vi "SVPO TDMS Write SGL Array (N Ch 1 Info).vi"(0 "tdms file":refnum<k34>, 1 "write channel properties? (T)":bool=TRUE, 5 "group name in":string="Waveform", 7 "channel names in":string[](array[string]), 9 "scaled signals [EU]":sgl[][](array[numeric]), 11 "sampling rate [Hz]":dbl=1.0, 12 "unit label":string) -> (4 "tdms file out":refnum<k34>, 6 "group name out":string, 8 "channel names out":string[](array[string]))   [LabVIEW 2017]
doc: "Writes single-precision waveform or scaled array data to the specified .tdms file in a format specific to the polymorphic instance. Use this VI on embedded targets that have limited computational resources. Wire data to the <B>scaled signal [EU]</B> input to determine the polymorphic instance to use or manually select the instance."
uses:
  <vilib>/addons/_NISVFA/_Shared subVIs/Controls/svc_X-Axis Units.ctl
  <vilib>/addons/_NISVFA/_Shared subVIs/Controls/NI Channel Properties.ctl
  <vilib>/addons/_NISVFA/_Shared subVIs/Controls/LV Datatypes.ctl
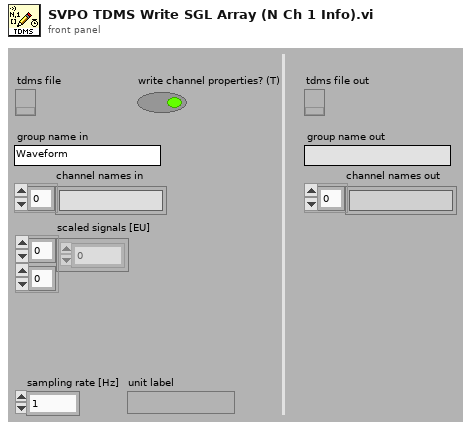
[diagram p1: front panel]
types:
  T1 = typedef "NI Channel Properties.ctl" = u16
  T2 = typedef "LV Datatypes.ctl" = i32
  T3 = typedef "svc_X-Axis Units.ctl" = u16
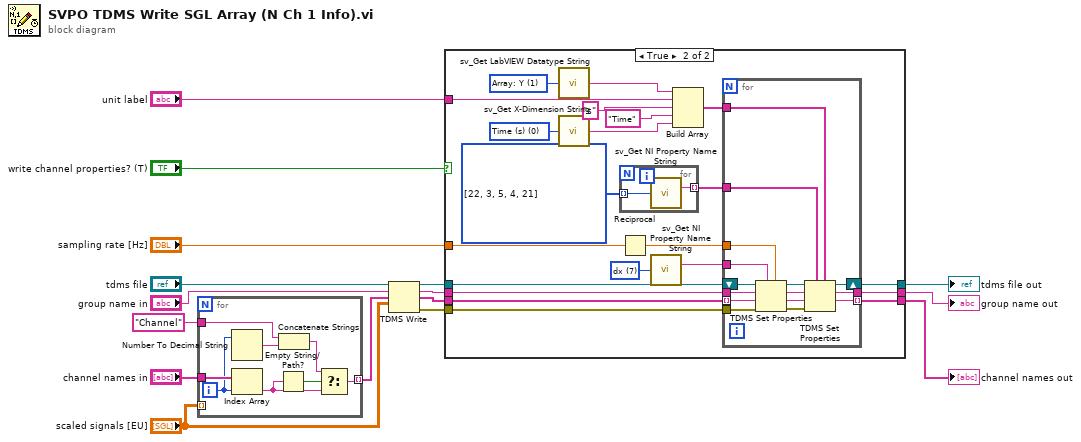
[diagram p0: block diagram]
diagram:
  n1 = for {
    tunnel: "channel names in" -> [w24]
    tunnel: [w23] -> w6 mode=indexing
    tunnel: "Channel" ("string") -> [w17]
    tunnel: "scaled signals [EU]" -> [_] mode=indexing
    i -> [w20]
    n2 = Number To Decimal String(number=w20) -> (decimal integer string=w19:string)  [unwired: 1 in]
    n3 = Index Array(array=w24, index=w20) -> (element=w21:string)
    n4 = Empty String/Path?(string/path=w21) -> (empty?=w22:bool)
    n5 = Concatenate Strings(w17, w19) -> (w18:string)
    n6 = Select(t=w18, s=w22, f=w21) -> (s? t:f=w23:string)
  }
  n7 = TDMS Write(0:"tdms file", 5:"group name in", 7:w6, 9:"scaled signals [EU]") -> (4:w15:refnum<k34>, 6:w13:string, 8:w12:string[], 15:w1:errorcluster)  [unwired: 2 in]
  n8 = case shown="True" "write channel properties? (T)" {
    tunnel: [w27 w41] -> w10
    tunnel: w12 -> [w25 w46]
    tunnel: w13 -> [w26 w45]
    tunnel: w15 -> [w27 w44]
    tunnel: [w26 w48] -> w9
    tunnel: [w25 w42] -> w4
    tunnel: "sampling rate [Hz]" -> [_ w38]
    tunnel: "unit label" -> [_ w34]
    tunnel: w1 -> [_ w36]
    frame False {
    }
    frame True {
      w28 = T1[] [22, 3, 5, 4, 21] items=["Channel name", "Channel description", "Y-axis label", "Y-axis unit string", "X-axis label", "X-axis unit string", "x0", "dx", "Number of samples", "X channel", "Filter settled", "dB reference", "Window", "Window parameter", "Window size", "FFT size", "Peak units", "Spectrum type", "Magnitude scale", "Spectral density", "Sensor sensitivity (mV/EU)", "X-axis domain", "LabVIEW datatype"]
      w47 = T2 1 items=["String"=-2, "Boolean"=-1, "Scalar: y"=0, "Array: Y"=1, "Waveform: t0, dt, Y, variant"=2, "Cluster: x0, dx, Y"=3, "Cluster: X, Y"=4, "Waterfall"=5, "Colormap"=6] ("LabVIEW datatype")
      w39 = T1 7 items=["Channel name", "Channel description", "Y-axis label", "Y-axis unit string", "X-axis label", "X-axis unit string", "x0", "dx", "Number of samples", "X channel", "Filter settled", "dB reference", "Window", "Window parameter", "Window size", "FFT size", "Peak units", "Spectrum type", "Magnitude scale", "Spectral density", "Sensor sensitivity (mV/EU)", "X-axis dimension", "LabVIEW datatype", "Function type", "Function subtype"] ("property")
      w43 = T3 0 items=["Time (s)"=0, "Frequency-CB (Hz)"=1, "Frequency-CPB (Hz)"=1248, "Frequency-Arbitrary (Hz)"=2357, "Quefrency (s)"=2, "Revolutions (rev)"=3, "Order"=4, "Speed (RPM)"=11, "Speed (rad/s)"=21, "Index"=65535] ("x-axis units")
      n9 = call <vilib>:"sv_Get LabVIEW Datatype String.vi"("LabVIEW datatype"=w47) -> ("datatype string"=w35:string)  [unwired: 4 in]
      n10 = call <vilib>:"sv_Get X-Dimension String.vi"("x-axis units"=w43) -> ("x-domain string"=w31:string)  [unwired: 4 in]
      n11 = for {
        tunnel: [w50] -> w29 mode=indexing
        tunnel: w28 -> [w49] mode=indexing
        n12 = call <vilib>:"sv_Get NI Property Name String.vi"("property"=w49) -> ("TDMS property name"=w50:string)  [unwired: 13 in, 1 out]
      }
      n13 = Reciprocal(x=w38) -> (1/x=w37:dbl)
      n14 = call <vilib>:"sv_Get NI Property Name String.vi"("property"=w39) -> ("TDMS property name"=w40:string)  [unwired: 13 in, 1 out]
      n15 = Build Array(w35, w34, "s" ("group name"), "Time" ("channel name"), w31) -> (w30:string[])
      n16 = for {
        tunnel: [w65] -> w48
        tunnel: w46 -> [w52] mode=indexing
        tunnel: w45 -> [w62]
        shift-right: [w64] -> w41
        shift-left: w44 -> [w63]
        tunnel: [w51] -> w42 mode=indexing
        tunnel: w40 -> [w61]
        tunnel: w37 -> [w60]
        tunnel: w36 -> [w59]
        tunnel: w30 -> [w54]
        tunnel: w29 -> [w53]
        n17 = TDMS Set Properties(5:w60, 7:w61, 8:w59, 9:w52, 10:w62, 11:w63) -> (0:w58:errorcluster, 1:w57:string, 2:w56:string, 3:w55:refnum<k34>)
        n18 = TDMS Set Properties(5:w54, 7:w53, 8:w58, 9:w57, 10:w56, 11:w55) -> (1:w51:string, 2:w65:string, 3:w64:refnum<k34>)  [unwired: 1 out]
      }
    }
  }
  "tdms file out" <- w10
  "group name out" <- w9
  "channel names out" <- w4
